vi "Extend.vi"(5 "Goal":dbl[](array[numeric]), 6 "Step":dbl, 7 "Initial State":dbl[](array[numeric]), 8 "enemy_robots":T1[](array[typedef]), 9 "Robot in":T1={"id"=0, "function"=enum."Attacker", "x"=0.0, "y"=0.0, "orientation"=0.0, "v_tangent"=0.0, "v_normal"=0.0, "v_ang"=0.0, "kick_x"=0.0, "kick_z"=0.0, "dribble"=FALSE, "Timestamp"=timestamp(0 s since 1904-01-01), "dest_x"=0.0, "dest_y"=0.0, "dest_orientation"=0.0, "estimatives"={"est_v_tangent"=0.0, "est_v_normal"=0.0, "est_vx"=0.0, "est_vy"=0.0, "Pos Robot Est"=[]}, "dest_x_kick"=0.0, "dest_y_kick"=0.0, "Gap Coord"=[], "States"=enum."GoToTangent", "Path "=[], "Path  Smooth"=[]}, 10 "Target":dbl[](array[numeric]), 11 "Nearest":dbl[](array[numeric])) -> (2 "New State":dbl[](array[numeric]))   [LabVIEW 2017]
uses:
  Core/AI Robot.ctl
  Intel/Functions Enum.ctl
  Intel/AttackerStates.ctl
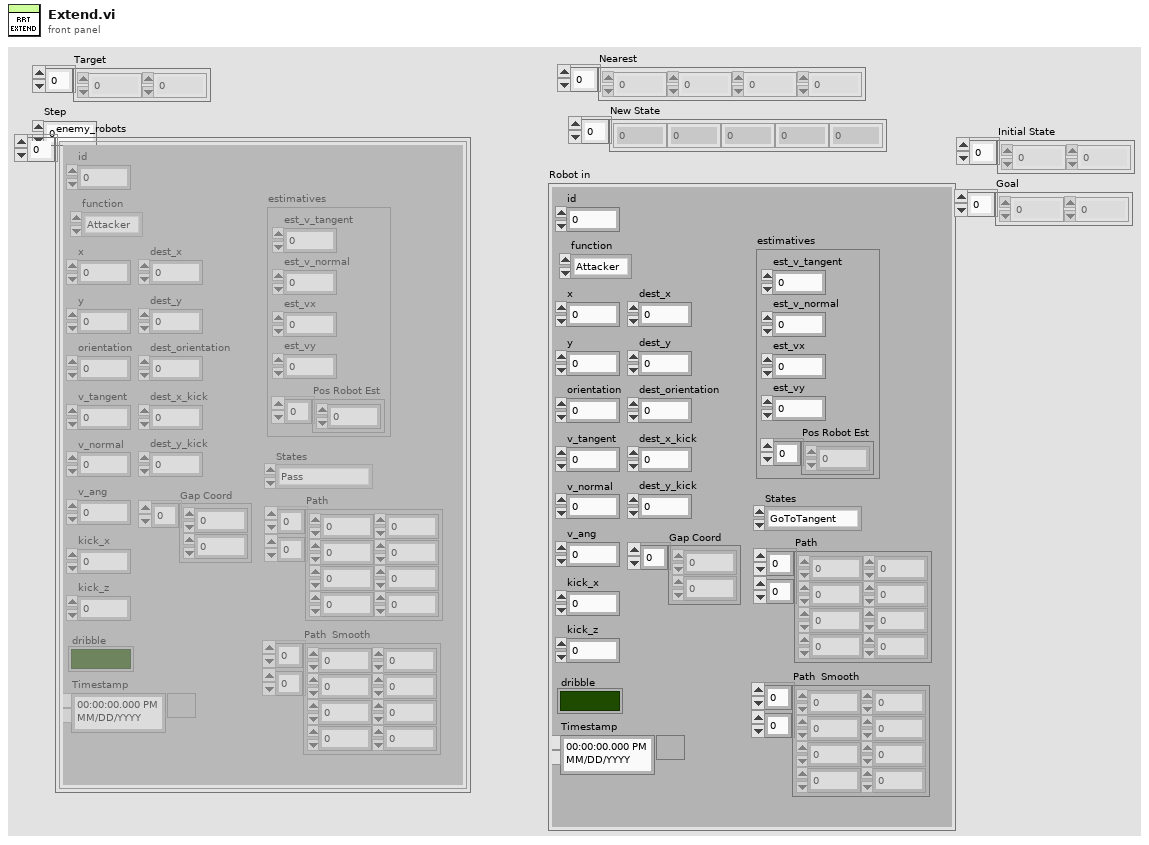
[diagram p1: front panel]
types:
  T1 = typedef "AI Robot.ctl" = cluster{"id":u32, "function":T2, "x":dbl, "y":dbl, "orientation":dbl, "v_tangent":dbl, "v_normal":dbl, "v_ang":dbl, "kick_x":dbl, "kick_z":dbl, "dribble":bool, "Timestamp":timestamp, "dest_x":dbl, "dest_y":dbl, "dest_orientation":dbl, "estimatives":cluster{"est_v_tangent":dbl, "est_v_normal":dbl, "est_vx":dbl, "est_vy":dbl, "Pos Robot Est":dbl[]}, "dest_x_kick":dbl, "dest_y_kick":dbl, "Gap Coord":dbl[], "States":T3, "Path ":dbl[][], "Path  Smooth":dbl[][]}
  T2 = typedef "Functions Enum.ctl" = enum16{"Attacker", "Goalie", "Defender", "Striker", "Goto 0", "Dummy", "Kicker", "ZigZag"}
  T3 = typedef "AttackerStates.ctl" = enum16{"Pass", "GoToTangent", "BallGetting", "GoToKick", ""}
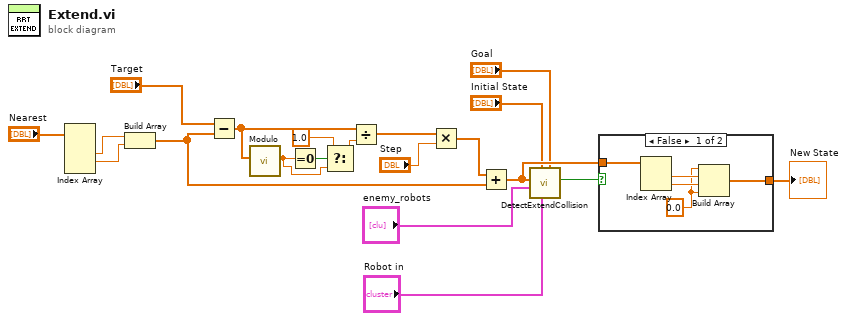
[diagram p0: block diagram]
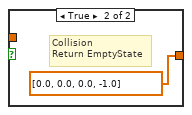
[diagram p2: hidden frame]
diagram:
  n1 = Index Array(array="Nearest") -> (element #2=w10:dbl, element #3=w9:dbl)  [unwired: 4 in, 2 out]
  n2 = Build Array(w10, w9) -> (w8:dbl[])
  n3 = Subtract(x="Target", y=w8) -> (x-y=w19:dbl[])
  n4 = call "Modulo.vi"("2D vector"=w19) -> ("Modulo"=w4:dbl)  [unwired: 10 in]
  n5 = Equal To 0?(x=w4) -> (x = 0?=w6:bool)
  n6 = Select(t=1.0, s=w6, f=w4) -> (s? t:f=w7:dbl)
  n7 = Divide(x=w19, y=w7) -> (x/y=w18:dbl[])
  n8 = Multiply(x=w18, y="Step") -> (x*y=w16:dbl[])
  n9 = Add(x=w16, y=w8) -> (x+y=w13:dbl[])
  n10 = call "DetectExtendCollision.vi"("Goal"="Goal", "Robot in"="Robot in", "Initial State"="Initial State", "enemy_robots"="enemy_robots", "Point"=w13) -> ("Collision"=w14:bool)  [unwired: 6 in]
  n11 = case shown="False" w14 {
    tunnel: [w21 dbl[] [0.0, 0.0, 0.0, -1.0] ("Nearest")] -> w12
    tunnel: w13 -> [w25 _]
    frame False {
      w22 = 0.0 ("element")
      n12 = Index Array(array=w25) -> (element #1=w24:dbl, element #2=w23:dbl)  [unwired: 2 in]
      n13 = Build Array(w22, w24, w23, w22) -> (w21:dbl[])
    }
    frame True {
      # "Collision\nReturn EmptyState"
    }
  }
  "New State" <- w12
